vi "GetDataFormat.vi"(1 "IOSource":T2, 5 "error in":errorcluster) -> (12 "Header out":T1={"Separator"="\t", "Remarks"="", "NDim"=0}, 13 "Names out":string[](array[string]), 14 "DataOK":bool, 15 "Found Header":bool, 16 "Data Type":i32, 17 "NData":i32, 18 "Sample Time":dbl format="%.10f", 19 "error out":errorcluster)   [LabVIEW 2020]
doc: "This VI checks the format of a data file. Sub-VI for Show_Save_Load_XY_Data.vi. See separate manual GCSData User SM146E.pdf and control descriptions in the diagram for more information."
panel:
  # "This vi checks the format of a data file. See separate manual \"GCSData User SM146E.pdf\"  and control descriptions in the \ndiagram for more information."
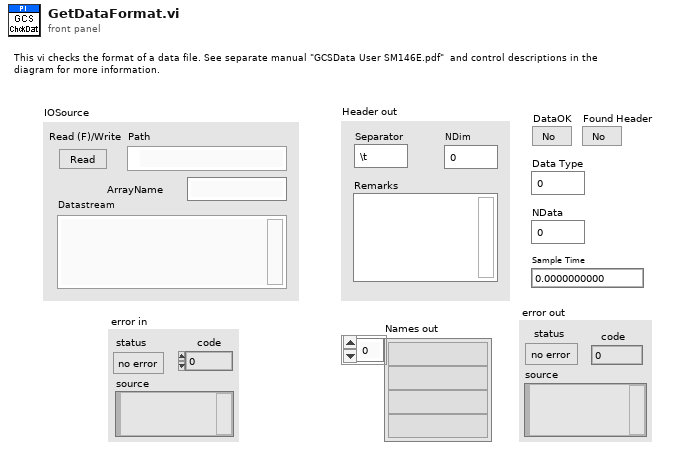
[diagram p1: front panel]
types:
  T1 = cluster{"Separator":string, "Remarks":string, "NDim":i32}
  T2 = cluster{"Read (F)/Write":bool, "Path":path, "Datastream":string, "ArrayName":string}
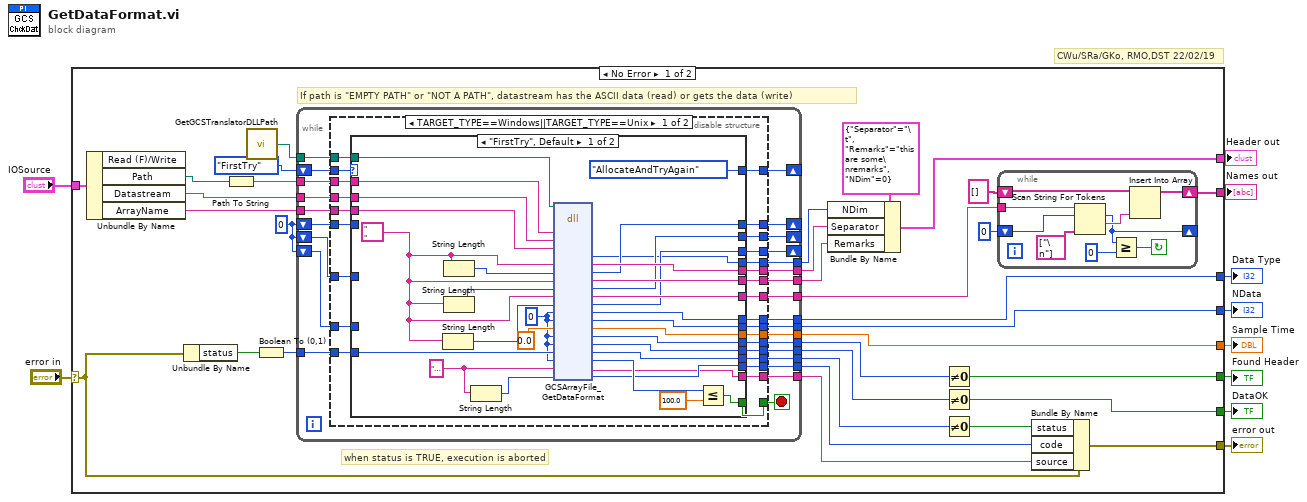
[diagram p0: block diagram]
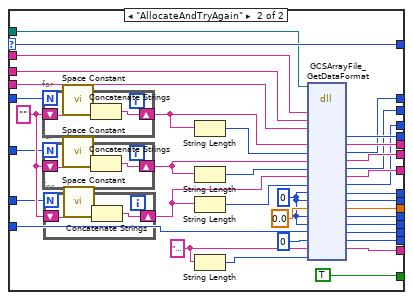
[diagram p2: hidden frame]
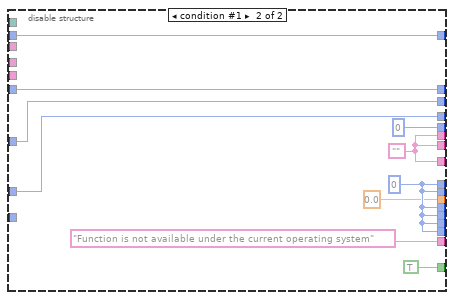
[diagram p3: hidden frame]
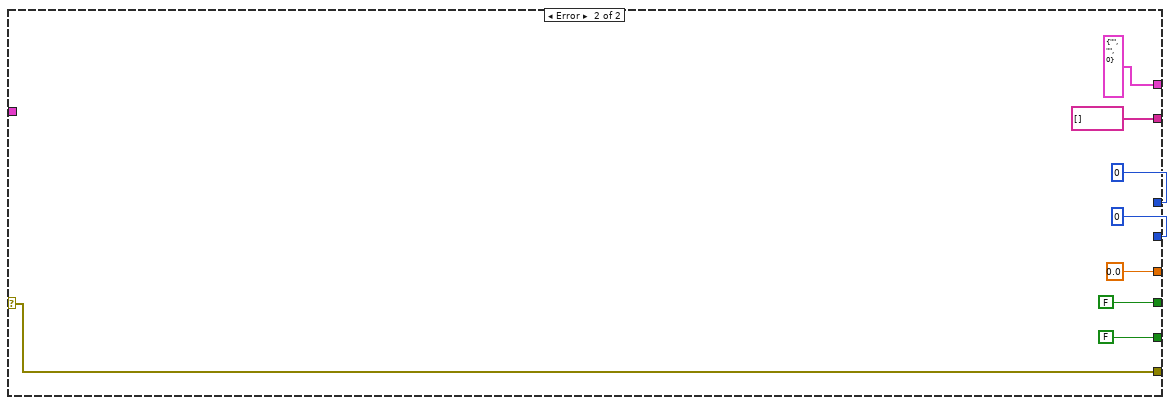
[diagram p4: hidden frame]
diagram:
  # "CWu/SRa/GKo, RMO,DST 22/02/19"
  n1 = case shown="No Error" "error in" {
    selector: "error in" -> [w11 w192]
    tunnel: [w41 T1 {"Separator"="", "Remarks"="", "NDim"=0} ("Header Out 2")] -> w10
    tunnel: [w40 string[] []] -> w9
    tunnel: [w35 0.0 ("SampleTime")] -> w8
    tunnel: [w34 u32 0 ("NData")] -> w7
    tunnel: [w33 0 ("DataType")] -> w6
    tunnel: [w30 FALSE] -> w5
    tunnel: [w29 FALSE] -> w4
    tunnel: [w20 w192] -> w3
    tunnel: "IOSource" -> [w12 _]
    frame No Error {
      w19 = u32 0 ("SeparatorBufferSize")
      # "when status is TRUE, execution is aborted"
      # "If path is \"EMPTY PATH\" or \"NOT A PATH\", datastream has the ASCII data (read) or gets the data (write)"
      n2 = Unbundle By Name(w12) -> ("Path"=w15:path, "Datastream"=w14:string, "ArrayName"=w13:string)  [unwired: 1 out]
      n3 = Unbundle By Name(w11) -> ("status"=w16:bool)
      n4 = Path To String(path=w15) -> (string=w27:string)
      n5 = call "GetGCSTranslatorDLLPath.vi"() -> ("DLL path"=w17:path)  [unwired: 1 in]
      n6 = Boolean To (0,1)(Boolean=w16) -> (0, 1=w24:i16)
      n7 = while {
        tunnel: [w68] -> w18
        tunnel: [w67] -> w37
        tunnel: [w66] -> w36
        tunnel: [w65] -> w35
        tunnel: [w64] -> w34
        tunnel: [w63] -> w33
        tunnel: [w62] -> w32
        tunnel: [w61] -> w31
        tunnel: w14 -> [w60]
        tunnel: w13 -> [w59]
        tunnel: [w58] -> w28
        tunnel: w27 -> [w54]
        tunnel: [w57] -> w26
        shift-right: [w51] -> _
        shift-left: w19 -> [w50]
        shift-right: [w52] -> _
        shift-left: w19 -> [w49]
        shift-right: [w53] -> _
        shift-left: w19 -> [w48]
        tunnel: w24 -> [w47]
        tunnel: [w46] -> w22
        tunnel: [w45] -> w21
        shift-right: [w44] -> _
        shift-left: enum16{"FirstTry", "AllocateAndTryAgain"}."FirstTry" -> [w56]
        tunnel: w17 -> [w43]
        stop <- w55 stop-if-true
        n8 = disable-structure shown="TARGET_TYPE==Windows||TARGET_TYPE==Unix" {
          disable-tunnel: [w94 u32 0 ("NDim")] -> w68
          disable-tunnel: [w93 w174] -> w67
          disable-tunnel: [w92 w174] -> w66
          disable-tunnel: [w91 0.0 ("SampleTime")] -> w65
          disable-tunnel: [w90 w176] -> w64
          disable-tunnel: [w89 w176] -> w63
          disable-tunnel: [w88 w176] -> w62
          disable-tunnel: [w87 w176] -> w61
          disable-tunnel: w60 -> [w86 _]
          disable-tunnel: w59 -> [w85 _]
          disable-tunnel: [w84 w176] -> w58
          disable-tunnel: [w83 w174] -> w57
          disable-tunnel: w56 -> [w82 w181]
          disable-tunnel: [w81 TRUE] -> w55
          disable-tunnel: w54 -> [w80 _]
          disable-tunnel: [w79 w178] -> w53
          disable-tunnel: [w78 w179] -> w52
          disable-tunnel: [w77 w182] -> w51
          disable-tunnel: w50 -> [w76 w182]
          disable-tunnel: w49 -> [w75 w179]
          disable-tunnel: w48 -> [w74 w178]
          disable-tunnel: w47 -> [w73 _]
          disable-tunnel: [w72 w176] -> w46
          disable-tunnel: [w71 "Function is not available under the current operating system" ("errorsource")] -> w45
          disable-tunnel: [w70 w181] -> w44
          disable-tunnel: w43 -> [w69 _]
          frame condition #0 (active) {
            n9 = case shown="\"FirstTry\", Default" w82 {
              selector: w82 -> [_ w132]
              tunnel: [w107 w163] -> w94
              tunnel: [w119 w162] -> w93
              tunnel: [w118 w161] -> w92
              tunnel: [w111 w160] -> w91
              tunnel: [w112 w159] -> w90
              tunnel: [w113 w158] -> w89
              tunnel: [w110 w157] -> w88
              tunnel: [w109 w156] -> w87
              tunnel: w86 -> [w122 w150]
              tunnel: w85 -> [w120 w149]
              tunnel: [w108 w145] -> w84
              tunnel: [w117 w144] -> w83
              tunnel: [w102 TRUE] -> w81
              tunnel: w80 -> [w121 w133]
              tunnel: [w116 w128] -> w79
              tunnel: [w115 w129] -> w78
              tunnel: [w114 w130] -> w77
              tunnel: w76 -> [_ w131]
              tunnel: w75 -> [_ w142]
              tunnel: w74 -> [_ w141]
              tunnel: w73 -> [w105 w135]
              tunnel: [w101 w139] -> w72
              tunnel: [w100 w140] -> w71
              tunnel: [enum16{"FirstTry", "AllocateAndTryAgain"}."AllocateAndTryAgain" w132] -> w70
              tunnel: w69 -> [w95 w127]
              frame "FirstTry", Default {
                w97 = "                                                                                                                                                  "
                w106 = "                               "
                w99 = u8 0 ("DataOK")
                n10 = String Length(string=w106) -> (length=w124:i32)
                n11 = String Length(string=w106) -> (length=w126:i32)
                n12 = String Length(string=w106) -> (length=w125:i32)
                n13 = String Length(string=w97) -> (length=w98:i32)
                n14 = dll-call lib="T:/Entwicklung/HostSoftware/LabVIEW/GCSDrivers/source/GCS2LabVIEW/Low Level/GCSTranslator.dll" fn="GCSArrayFile_GetDataFormat"(path in=w95, "Path"=w121, "DataStream"=w122, "ArrayName"=w120, "Separator"=w106, "SeparatorBufferSize"=w126, "Remarks"=w106, "RemarksBufferSize"=w125, "ArrayColumnNames"=w106, "ArrayColumnNameBufferSize"=w124, "DataType"=w99, "NData"=w99, "SampleTime"=0.0, "FoundHeader"=w99, "DataOK"=w99, "errorstatus"=w105, "errorcode"=w99, "errorsource"=w97, "errorsrcbuflen"=w98) -> ("NDim"=w107:u32, "Separator"=w119:string, "SeparatorBufferSize"=w114:u32, "Remarks"=w118:string, "RemarksBufferSize"=w115:u32, "ArrayColumnNames"=w117:string, "ArrayColumnNameBufferSize"=w116:u32, "DataType"=w113:i32, "NData"=w112:u32, "SampleTime"=w111:dbl, "FoundHeader"=w110:u8, "DataOK"=w109:u8, "errorstatus"=w108:u8, "errorcode"=w103:i32, "errorsource"=w100:string, "errorsrcbuflen"=w101:u32)  [unwired: 5 in, 4 out]
                n15 = Less Or Equal?(x=w103, y=100.0) -> (x <= y?=w102:bool)
              }
              frame "AllocateAndTryAgain" {
                w138 = "                                                                                                                                                  "
                w147 = ""
                w151 = u8 0 ("DataOK")
                n16 = for {
                  N: w131 -> [_]
                  shift-right: [w165] -> w148
                  shift-left: w147 -> [w164]
                  n17 = call <vilib>:"Space Constant.vi"() -> ("String"=w166:string)
                  n18 = Concatenate Strings(w166, w164) -> (w165:string)
                }
                n19 = for {
                  N: w142 -> [_]
                  shift-right: [w168] -> w134
                  shift-left: w147 -> [w167]
                  n20 = call <vilib>:"Space Constant.vi"() -> ("String"=w169:string)
                  n21 = Concatenate Strings(w169, w167) -> (w168:string)
                }
                n22 = for {
                  N: w141 -> [_]
                  shift-right: [w171] -> w146
                  shift-left: w147 -> [w170]
                  n23 = call <vilib>:"Space Constant.vi"() -> ("String"=w172:string)
                  n24 = Concatenate Strings(w172, w170) -> (w171:string)
                }
                n25 = String Length(string=w148) -> (length=w155:i32)
                n26 = String Length(string=w134) -> (length=w154:i32)
                n27 = String Length(string=w146) -> (length=w153:i32)
                n28 = String Length(string=w138) -> (length=w137:i32)
                n29 = dll-call lib="T:/Entwicklung/HostSoftware/LabVIEW/GCSDrivers/source/GCS2LabVIEW/Low Level/GCSTranslator.dll" fn="GCSArrayFile_GetDataFormat"(path in=w127, "Path"=w133, "DataStream"=w150, "ArrayName"=w149, "Separator"=w148, "SeparatorBufferSize"=w155, "Remarks"=w134, "RemarksBufferSize"=w154, "ArrayColumnNames"=w146, "ArrayColumnNameBufferSize"=w153, "DataType"=w151, "NData"=w151, "SampleTime"=0.0, "FoundHeader"=w151, "DataOK"=w151, "errorstatus"=w135, "errorcode"=0, "errorsource"=w138, "errorsrcbuflen"=w137) -> ("NDim"=w163:u32, "Separator"=w162:string, "SeparatorBufferSize"=w130:u32, "Remarks"=w161:string, "RemarksBufferSize"=w129:u32, "ArrayColumnNames"=w144:string, "ArrayColumnNameBufferSize"=w128:u32, "DataType"=w158:i32, "NData"=w159:u32, "SampleTime"=w160:dbl, "FoundHeader"=w157:u8, "DataOK"=w156:u8, "errorstatus"=w145:u8, "errorcode"=w139:i32, "errorsource"=w140:string)  [unwired: 5 in, 5 out]
              }
            }
          }
          frame condition #1 {
            w174 = "" ("ArrayColumnNames")
            w176 = u8 0 ("DataOK")
          }
        }
      }
      n30 = Bundle By Name(cluster=T1 {"Separator"="\t", "Remarks"="this are some\nremarks", "NDim"=0} ("Header Out 2"), "NDim"=w18, "Separator"=w37, "Remarks"=w36) -> (w41:T1)
      n31 = Not Equal To 0?(x=w32) -> (x != 0?=w30:bool)
      n32 = Not Equal To 0?(x=w31) -> (x != 0?=w29:bool)
      n33 = Not Equal To 0?(x=w28) -> (x != 0?=w23:bool)
      n34 = while {
        shift-right: [w189] -> w40
        shift-left: string[] [] -> [w188]
        shift-right: [w185] -> _
        shift-left: 0 ("offset past token") -> [w186]
        tunnel: w26 -> [w184]
        stop <- w190 continue-if-true
        n35 = Scan String For Tokens(6:string[] ["\n"] ("delimiters (\\s,\\t,\\r,\\n)"), 8:w186, 9:w184) -> (1:w187:string, 2:w185:i32)  [unwired: 5 out]
        n36 = Greater Or Equal?(x=w185, y=0) -> (x >= y?=w190:bool)
        n37 = Insert Into Array(array=w188, new element=w187) -> (w189:string[])  [unwired: 1 in]
      }
      n38 = Bundle By Name(cluster=w11, "status"=w23, "code"=w22, "source"=w21) -> (w20:errorcluster)
    }
    frame Error {
    }
  }
  "error out" <- w3
  "Header out" <- w10
  "Names out" <- w9
  "Data Type" <- w6
  "NData" <- w7
  "Found Header" <- w5
  "DataOK" <- w4
  "Sample Time" <- w8
